vi "Short and Filter Table.vi"(5 "Sort By Ref":refnum<vi>, 6 "Headers":string[](array[string]), 7 "Filter String Ref":refnum<vi>, 8 "error in":errorcluster, 11 "Table Ref":refnum<vi>) -> (0 "error out":errorcluster, 3 "Sorted Table Data out":string[][](array[string]))   [LabVIEW 2025, in "Automotive Ethernet Bus Monitor UI.lvlib"]
doc: "Short and Filter the data based on the Short By and Filter Inputs, when this functionality is not paused."
uses:
  Automotive Ethernet Bus Monitor UI.lvlib
  Table_Filtering/Table_Filtering.lvlib
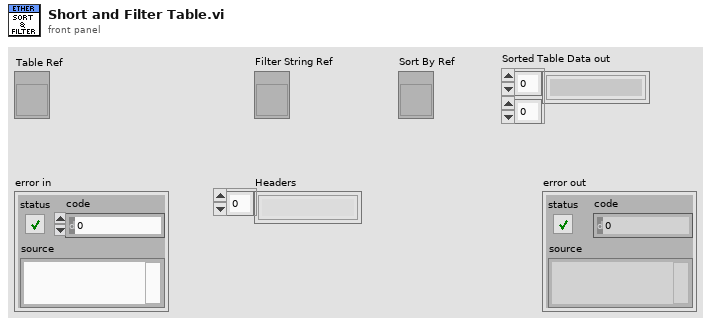
[diagram p1: front panel]
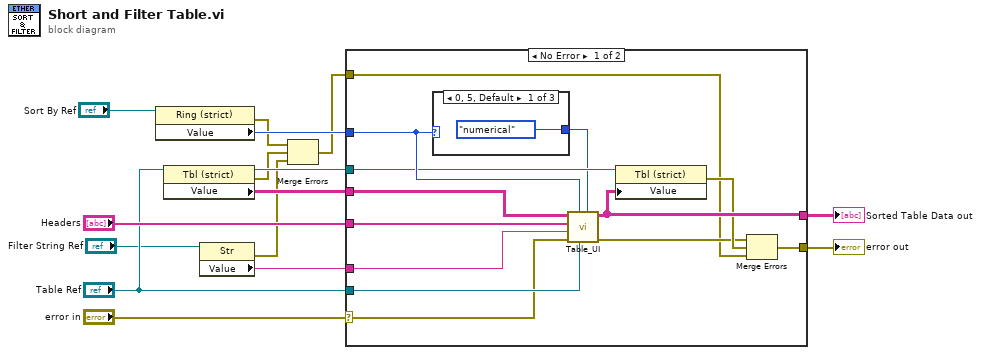
[diagram p0: block diagram]
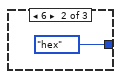
[diagram p2: hidden frame]
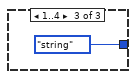
[diagram p3: hidden frame]
diagram:
  n1 = property class="Ring (strict)"(reference="Sort By Ref") -> (error out=w5:errorcluster, "Value"=w6:u16)  [unwired: 1 in, 1 out]
  n2 = property class="Tbl (strict)"(reference="Table Ref") -> (reference out=w10:refnum<vi>, error out=w3:errorcluster, "Value"=w12:string[][])  [unwired: 1 in]
  n3 = property class="Str"(reference="Filter String Ref") -> (error out=w4:errorcluster, "Value"=w7:string)  [unwired: 1 in, 1 out]
  n4 = Merge Errors(w5, w3, w4) -> (w1:errorcluster)
  n5 = case shown="No Error" "error in" {
    selector: "error in" -> [w26 w32]
    tunnel: w6 -> [w28 _]
    tunnel: w7 -> [w24 _]
    tunnel: "Headers" -> [w23 _]
    tunnel: [w22 w32] -> w2
    tunnel: "Table Ref" -> [w27 _]
    tunnel: [w25 w33] -> w11
    tunnel: w12 -> [w21 w33]
    tunnel: w10 -> [w20 _]
    tunnel: w1 -> [w16 _]
    frame No Error {
      n6 = case shown="0, 5, Default" w28 {
        tunnel: [enum16{"numerical", "hex", "string"}."numerical" ("Sort Type") enum16{"numerical", "hex", "string"}."hex" ("Sort Type") enum16{"numerical", "hex", "string"}."string" ("Sort Type")] -> w19
        frame 0, 5, Default {
        }
        frame 6 {
        }
        frame 1..4 {
        }
      }
      n7 = call "Table_UI.vi"("Sort Type"=w19, "Table Control"=w27, "Sort by"=w28, "error in"=w26, "Filter String"=w24, "Headers"=w23, "Unsorted Data"=w21) -> ("Error Out"=w17:errorcluster, "Table Control"=w25:string[][])  [unwired: 3 in]
      n8 = property class="Tbl (strict)"(reference=w20, "Value"=w25) -> (error out=w18:errorcluster)  [unwired: 1 in, 1 out]
      n9 = Merge Errors(w17, w18, w16) -> (w22:errorcluster)
    }
    frame Error {
    }
  }
  "error out" <- w2
  "Sorted Table Data out" <- w11
